vi "Write Device.vi"(8 "error in":errorcluster, 10 "Device":string, 11 "SLL in":refnum<class "SLL.lvclass">) -> (0 "error out":errorcluster, 3 "SLL out":refnum<class "SLL.lvclass">)   [LabVIEW 2023, in "SLL.lvlib" / "SLL.lvclass"]
uses:
  SLL.lvclass
  SLL.lvclass/SLL.ctl
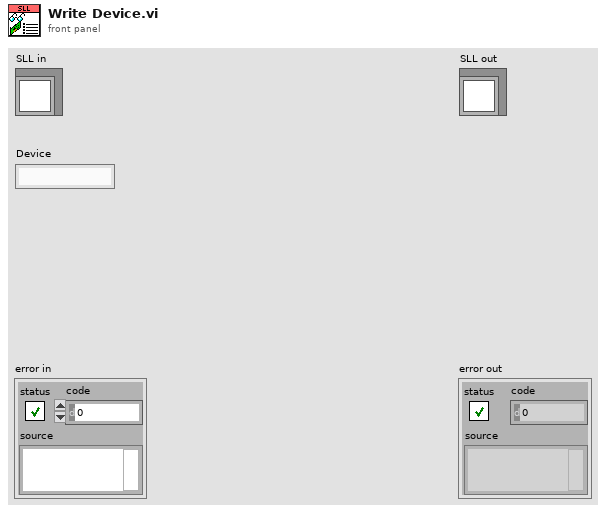
[diagram p1: front panel]
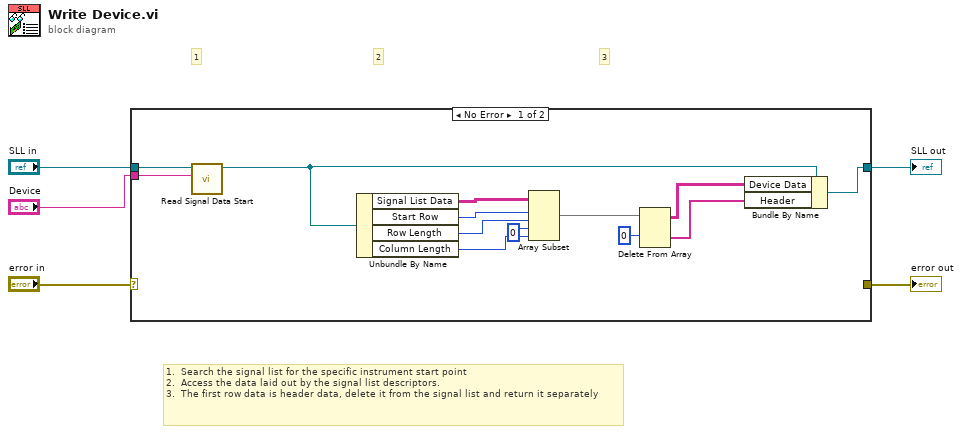
[diagram p0: block diagram]
diagram:
  # "1.  Search the signal list for the specific instrument start point\n2.  Access the data laid out by the signal list descriptors.\n3.  The first row data is header data, delete it from the signal list and return it separately"
  # "3"
  # "2"
  # "1"
  n1 = case shown="No Error" "error in" {
    selector: "error in" -> [_ w20]
    tunnel: [_ w20] -> w4
    tunnel: [w6 w19] -> w3
    tunnel: "SLL in" -> [w18 w19]
    tunnel: "Device" -> [w17 _]
    frame No Error {
      n2 = call "Read Signal Data Start.vi"("Device"=w17, "SLL in"=w18) -> ("SLL out"=w9:refnum<class "SLL.lvclass">)  [unwired: 8 in, 1 out]
      n3 = Unbundle By Name(w9) -> ("Signal List Data"=w16:string[][], "Start Row"=w15:i32, "Row Length"=w14:i32, "Column Length"=w13:i32)
      n4 = Array Subset(array=w16, index (row)=w15, length (row)=w14, index (col)=0 ("index"), length (col)=w13) -> (w11:string[][])
      n5 = Delete From Array(array=w11, index (row)=0) -> (deleted portion=w7:string[], array with subset deleted=w8:string[][])  [unwired: 2 in]
      n6 = Bundle By Name(cluster=w9, "Device Data"=w8, "Header"=w7) -> (w6:refnum<class "SLL.lvclass">)
    }
    frame Error {
    }
  }
  "error out" <- w4
  "SLL out" <- w3
